vi "TWM Client Cmd Identify.vi"(5 "timeout [ms]":i32=5000, 7 "end of packet key":string="TWM:command:EndOfPacket", 8 "error in":errorcluster, 11 "handle":i32) -> (0 "error out":errorcluster, 1 "aux idns":string[](array[string]), 2 "channel idns":string[](array[string]), 3 "handle out":i32)   [LabVIEW 2013, in "TWM Client.lvlib"]
doc: "Write Identify command packet to TWM server. Wait for answer. Parse and return data."
uses:
  TWM Client.lvlib
  octave/infolib.lvlibp/Private/Get matrix polymorph parts/Get 1D String.vi
  <vilib>/Utility/error.llb/Error Cluster From Error Code.vi
  <vilib>/ErrorRing/Error Ring.xnode
  octave/infolib.lvlibp
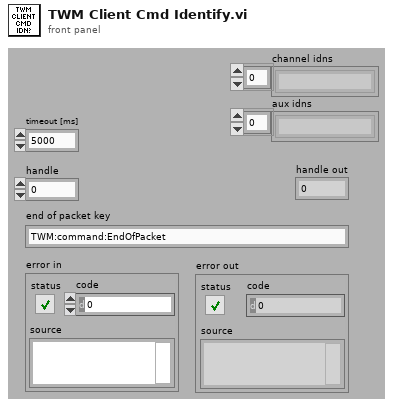
[diagram p1: front panel]
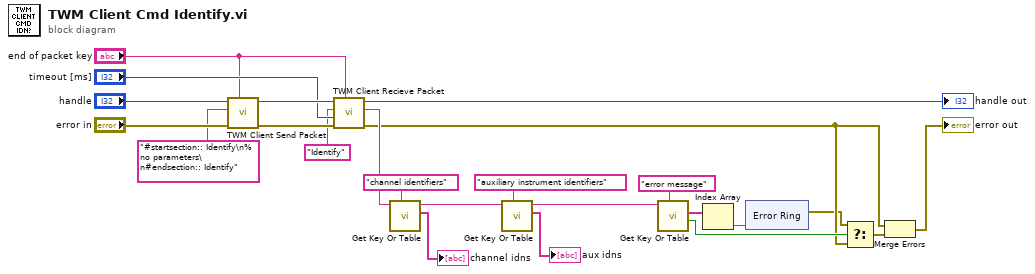
[diagram p0: block diagram]
diagram:
  n1 = call "TWM Client Send Packet.vi"("end of packet key"="end of packet key", "error in"="error in", "command string"="#startsection:: Identify\n% no parameters\n#endsection:: Identify", "handle"="handle") -> ("error out"=w21:errorcluster, "handle out"=w20:i32)  [unwired: 6 in]
  n2 = call "TWM Client Recieve Packet.vi"("end of packet key"="end of packet key", "error in"=w21, "timeout [ms] (5000 ms)"="timeout [ms]", "message header (empty)"="Identify", "handle in"=w20) -> ("error out"=w2:errorcluster, "message data"=w15:string, "handle out"=→"handle out":i32)  [unwired: 4 in]
  n3 = call-poly "Get Key Or Table.vi"("key description"="channel identifiers", "info data"=w15) -> ("value"=→"channel idns":string[], "info data out"=w12:string)  [unwired: 6 in, 2 out]
  n4 = call-poly "Get Key Or Table.vi"("key description"="auxiliary instrument identifiers", "info data"=w12) -> ("value"=→"aux idns":string[], "info data out"=w8:string)  [unwired: 6 in, 2 out]
  n5 = call-poly "Get Key Or Table.vi"("key description"="error message", "info data"=w8) -> ("found?"=w5:bool, "value"=w4:string[])  [unwired: 6 in, 2 out]
  n6 = Index Array(array=w4) -> (element=w3:string)  [unwired: 1 in]
  n7 = xnode "Error Ring"("parameter 0"=w3) -> ("error out"=w1:errorcluster)
  n8 = Select(t=w1, s=w5, f=w2) -> (s? t:f=w7:errorcluster)
  n9 = Merge Errors(w2, w7) -> (→"error out":errorcluster)
